vi "save_configuration.vi"(8 "error in (no error)":errorcluster, 10 "config cluster variant in (data type)":variant, 11 "path":path) -> (0 "error out":errorcluster)   [LabVIEW 2010]
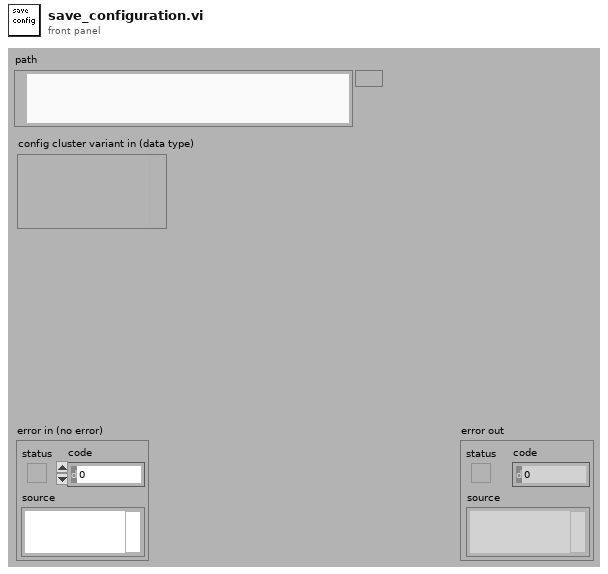
[diagram p1: front panel]
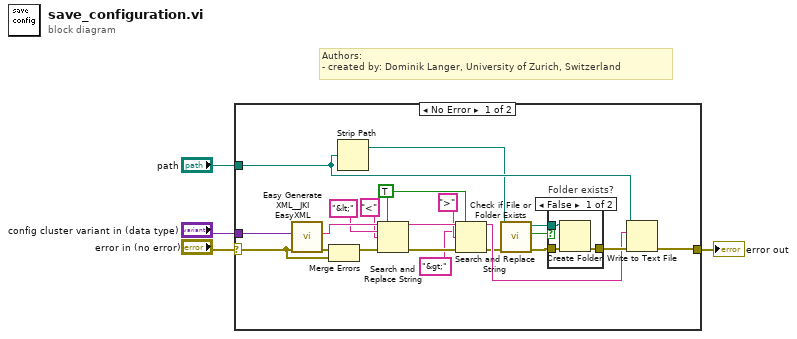
[diagram p0: block diagram]
diagram:
  # "Authors: \n- created by: Dominik Langer, University of Zurich, Switzerland"
  n1 = case shown="No Error" "error in (no error)" {
    selector: "error in (no error)" -> [w17 w30]
    tunnel: [w25 w30] -> w3
    tunnel: "config cluster variant in (data type)" -> [w24 _]
    tunnel: "path" -> [w23 _]
    frame No Error {
      w5 = TRUE ("replace all? (F)")
      n2 = call <vilib>:"Easy Generate XML__JKI EasyXML.vi"("error in (no error)"=w17, "LabVIEW Data"=w24) -> ("error out"=w16:errorcluster, "XML String"=w14:string)  [unwired: 1 in, 7 out]
      n3 = Merge Errors(w16, w17) -> (w15:errorcluster)
      n4 = Strip Path(path=w23) -> (stripped path=w21:path)  [unwired: 1 out]
      n5 = Search and Replace String(replace all?=w5, input string=w14, search string="&lt;", replace string="<" ("replace string (\"\")"), error in=w15) -> (result string=w11:string, error out=w8:errorcluster)  [unwired: 3 in, 2 out]
      n6 = Search and Replace String(replace all?=w5, input string=w11, search string="&gt;", replace string=">" ("replace string (\"\")"), error in=w8) -> (result string=w10:string, error out=w9:errorcluster)  [unwired: 3 in, 2 out]
      n7 = call <vilib>:"Check if File or Folder Exists.vi"("error in (no error)"=w9, "path"=w21) -> ("error out"=w18:errorcluster, "file or folder exists?"=w19:bool, "dup path"=w20:path)  [unwired: 7 out]
      n8 = case "Folder exists?" shown="False" w19 {
        tunnel: [w28 w29] -> w22
        tunnel: w20 -> [w27 _]
        tunnel: w18 -> [w26 w29]
        frame False {
          n9 = Create Folder(path (use dialog)=w27, error in=w26) -> (error out=w28:errorcluster)  [unwired: 3 out]
        }
        frame True {
        }
      }
      n10 = Write to Text File(file (use dialog)=w23, text=w10, error in=w22) -> (error out=w25:errorcluster)  [unwired: 3 out]
    }
    frame Error {
    }
  }
  "error out" <- w3
